vi "读取产品参数信息-CCD3CCD4.vi"(8 "错误输入（无错误）":errorcluster, 11 "LoadProductName":string) -> (0 "错误输出":errorcluster)   [LabVIEW 2017]
uses:
  Global System.vi
panel:
  out "添加的路径":path
  out "连接的字符串":string
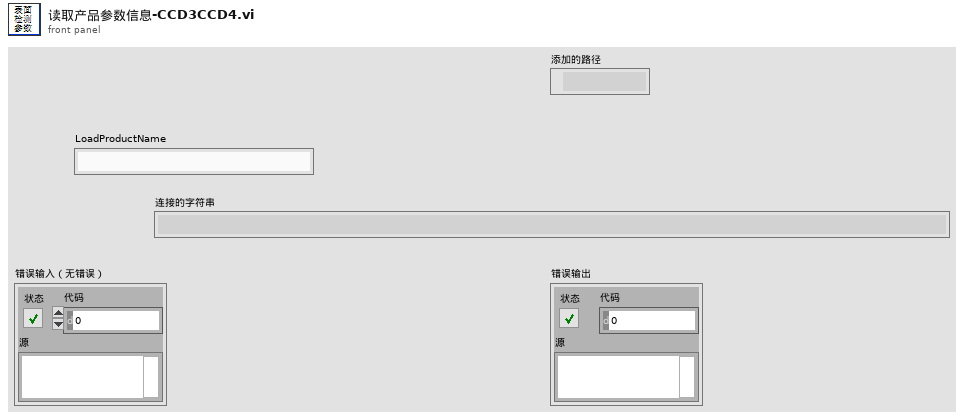
[diagram p1: front panel]
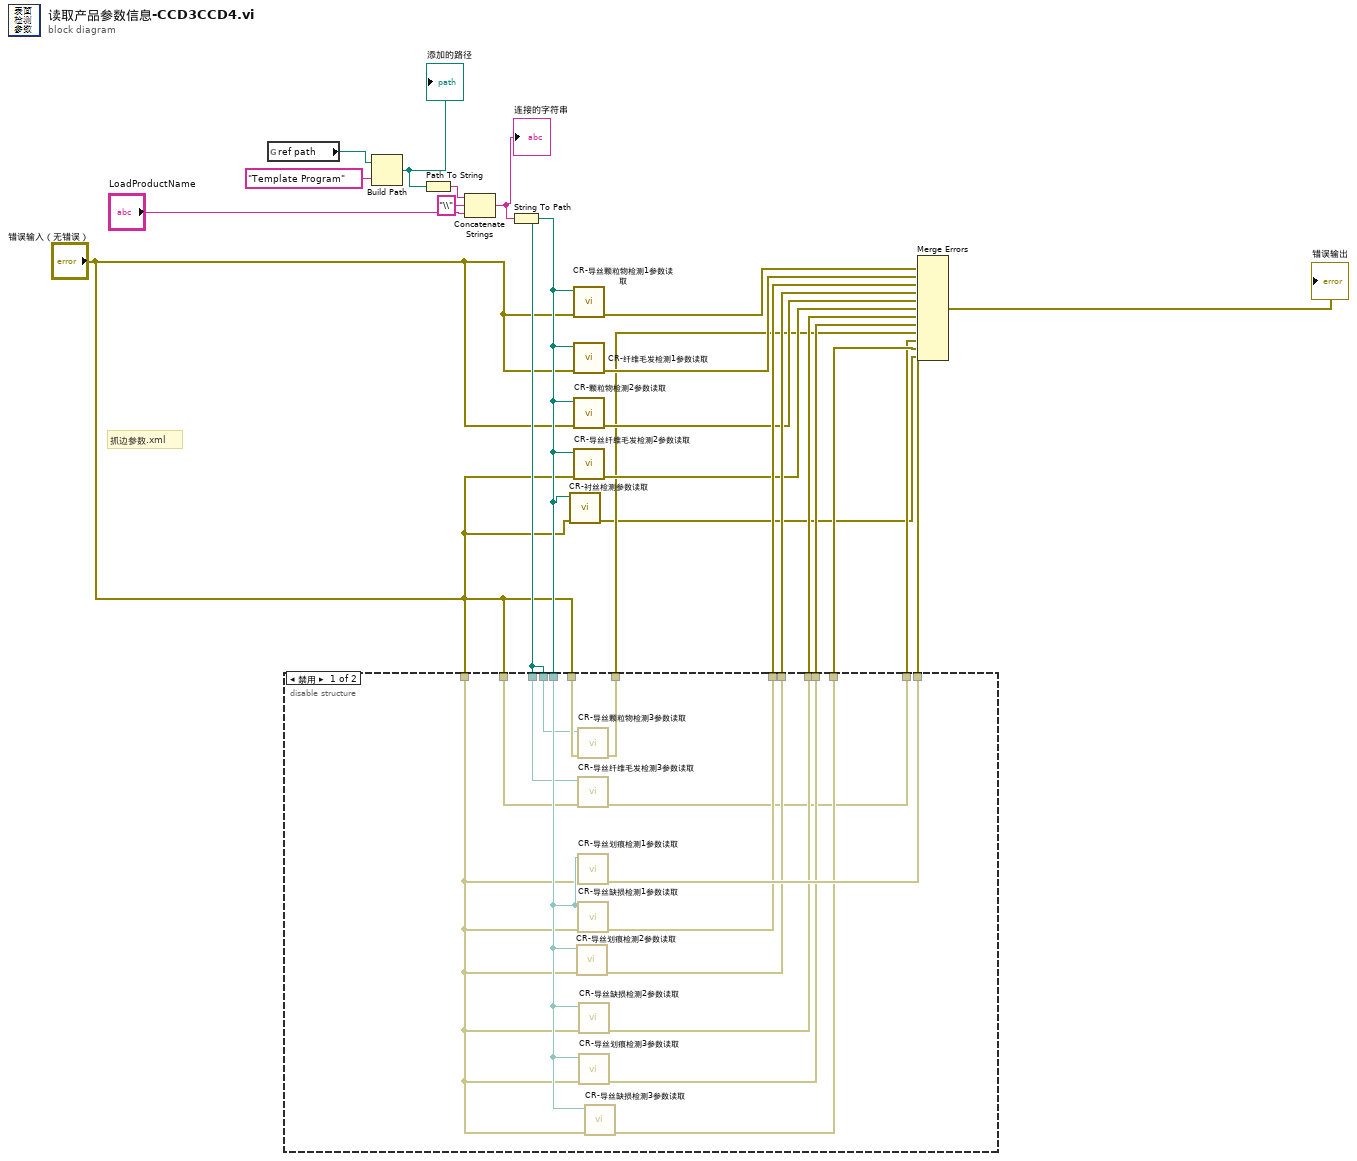
[diagram p0: block diagram]
diagram:
  # "抓边参数.xml"
  n1 = global read "Global System.vi" "ref path"() -> (w23:path)
  n2 = Build Path(base path=w23, name or relative path="Template Program" ("名称或相对路径")) -> (appended path=w21:path)
  "添加的路径" <- w21
  n3 = Path To String(path=w21) -> (string=w20:string)
  n4 = Concatenate Strings(w20, "\\" ("字符串"), "LoadProductName") -> (w17:string)
  "连接的字符串" <- w17
  n5 = String To Path(string=w17) -> (path=w3:path)
  n6 = disable-structure shown="禁用" {
    disable-tunnel: [w37 _] -> w16
    disable-tunnel: [w36 _] -> w12
    disable-tunnel: [w35 _] -> w11
    disable-tunnel: w3 -> [w34 _]
    disable-tunnel: "错误输入（无错误）" -> [w33 _]
    disable-tunnel: [w32 _] -> w8
    disable-tunnel: [w31 _] -> w7
    disable-tunnel: [w30 _] -> w6
    disable-tunnel: "错误输入（无错误）" -> [w29 _]
    disable-tunnel: w3 -> [w28 _]
    disable-tunnel: "错误输入（无错误）" -> [w27 _]
    disable-tunnel: w3 -> [w26 _]
    disable-tunnel: [w25 _] -> w5
    disable-tunnel: [w24 _] -> w4
    frame Disabled {
      n7 = call "CR-导丝划痕检测2参数读取.vi"("error in (no error)"=w33, "基路径"=w34) -> ("error out"=w35:errorcluster)  [unwired: 6 in, 2 out]
      n8 = call "CR-导丝颗粒物检测3参数读取.vi"("error in (no error)"=w27, "基路径"=w26) -> ("error out"=w24:errorcluster)  [unwired: 6 in, 2 out]
      n9 = call "CR-导丝纤维毛发检测3参数读取.vi"("error in (no error)"=w29, "基路径"=w28) -> ("error out"=w25:errorcluster)  [unwired: 6 in, 2 out]
      n10 = call "CR-导丝划痕检测1参数读取.vi"("error in (no error)"=w33, "基路径"=w34) -> ("error out"=w37:errorcluster)  [unwired: 6 in, 2 out]
      n11 = call "CR-导丝缺损检测1参数读取.vi"("error in (no error)"=w33, "基路径"=w34) -> ("error out"=w36:errorcluster)  [unwired: 6 in, 2 out]
      n12 = call "CR-导丝缺损检测2参数读取.vi"("error in (no error)"=w33, "基路径"=w34) -> ("error out"=w32:errorcluster)  [unwired: 6 in, 2 out]
      n13 = call "CR-导丝划痕检测3参数读取.vi"("error in (no error)"=w33, "基路径"=w34) -> ("error out"=w31:errorcluster)  [unwired: 6 in, 2 out]
      n14 = call "CR-导丝缺损检测3参数读取.vi"("error in (no error)"=w33, "基路径"=w34) -> ("error out"=w30:errorcluster)  [unwired: 6 in, 2 out]
    }
    frame Enabled {
    }
  }
  n15 = call "CR-衬丝检测参数读取.vi"("error in (no error)"="错误输入（无错误）", "基路径"=w3) -> ("error out"=w1:errorcluster)  [unwired: 5 in, 3 out]
  n16 = call "CR-导丝颗粒物检测1参数读取.vi"("error in (no error)"="错误输入（无错误）", "基路径"=w3) -> ("error out"=w14:errorcluster)  [unwired: 6 in, 2 out]
  n17 = call "CR-纤维毛发检测1参数读取.vi"("error in (no error)"="错误输入（无错误）", "基路径"=w3) -> ("error out"=w13:errorcluster)  [unwired: 6 in, 2 out]
  n18 = call "CR-颗粒物检测2参数读取.vi"("error in (no error)"="错误输入（无错误）", "基路径"=w3) -> ("error out"=w10:errorcluster)  [unwired: 6 in, 2 out]
  n19 = call "CR-导丝纤维毛发检测2参数读取.vi"("error in (no error)"="错误输入（无错误）", "基路径"=w3) -> ("error out"=w9:errorcluster)  [unwired: 6 in, 2 out]
  n20 = Merge Errors(w16, w14, w13, w12, w11, w10, w9, w8, w7, w4, w5, w6, w1) -> (→"错误输出":errorcluster)
